vi "Is FIXSTR.vi"(11 "bytes":u8[](array[numeric])) -> (2 "Is FIXSTR?":bool, 3 "bytes":u8[](array[numeric]))   [LabVIEW 2020, in "wamplv.lvlib" / "MessagePack.lvclass"]
uses:
  MessagePack.lvclass
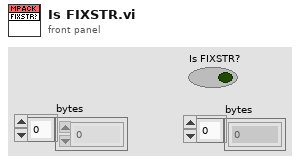
[diagram p1: front panel]
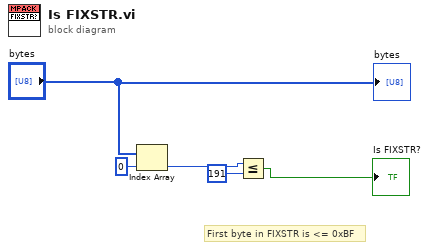
[diagram p0: block diagram]
diagram:
  # "First byte in FIXSTR is <= 0xBF"
  n1 = Index Array(array="bytes", index=0) -> (element=w3:u8)
  n2 = Less Or Equal?(x=w3, y=u8 191) -> (x <= y?=→"Is FIXSTR?":bool)
  "bytes" <- "bytes"
